vi "Map Child Elements.vi"(8 "error in":errorcluster, 10 "Address":i32[](array[numeric]), 11 "XML Document in":refnum<class "XML Document.lvclass">) -> (0 "error out":errorcluster, 3 "XML Document out":refnum<class "XML Document.lvclass">)   [LabVIEW 2014, in "XML Document.lvclass"]
uses:
  XML Document.lvclass
  Controls/Node Type.ctl
  Node_class/Node.lvclass
  <vilib>/xml/Close Reference(Node).vi
  <resource>/objmgr/DOMUserDefRef.rc
  Element_class/Element.lvclass
  Text Node_class/Text Node.lvclass
  Comment Node_class/Comment Node.lvclass
  <vilib>/xml/NI_XML.lvlib
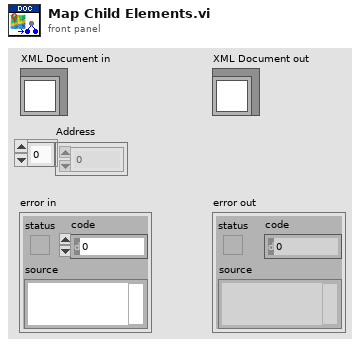
[diagram p1: front panel]
types:
  T1 = typedef "Node Type.ctl" = i32
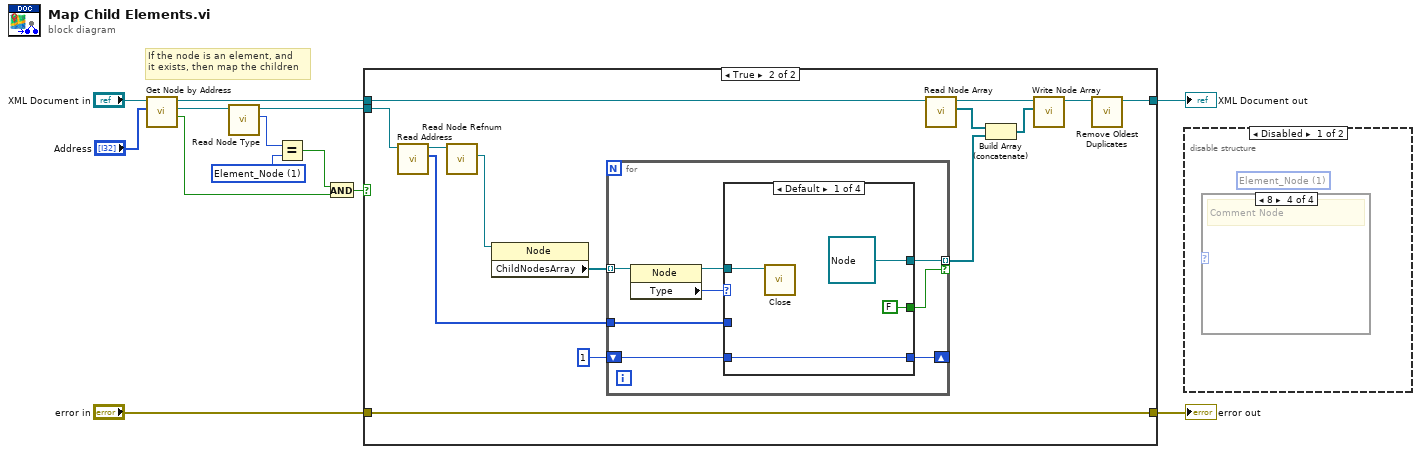
[diagram p0: block diagram]
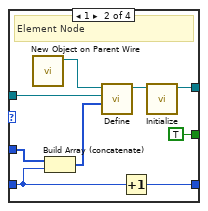
[diagram p7: hidden frame]
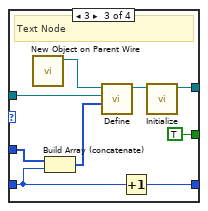
[diagram p8: hidden frame]
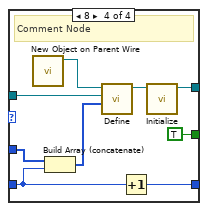
[diagram p9: hidden frame]
diagram:
  w4 = T1 1 items=["Element_Node"=1, "Attribute_Node"=2, "Text_Node"=3, "CDATASection_Node"=4, "EntityReference_Node"=5, "Entity_Node"=6, "ProcessingInstruction_Node"=7, "Comment_Node"=8, "Document_Node"=9, "DocumentType_Node"=10, "DocumentFragment_Node"=11, "Notation_Node"=12] ("y")
  # "If the node is an element, and\nit exists, then map the children"
  n1 = call "Get Node by Address.vi"("Address"="Address", "XML Document in"="XML Document in") -> ("Found?"=w3:bool, "Node.lvclass"=w9:refnum<class "Node.lvclass">, "XML Document out"=w10:refnum<class "XML Document.lvclass">)  [unwired: 6 in, 1 out]
  n2 = call-dynamic "Read Node Type.vi"("Node in"=w9) -> ("Node Type"=w5:T1, "Node out"=w6:refnum<class "Node.lvclass">)  [unwired: 8 in, 1 out]
  n3 = Equal?(x=w5, y=w4) -> (x = y?=w2:bool)
  n4 = And(x=w2, y=w3) -> (x .and. y?=w1:bool)
  n5 = case shown="True" w1 {
    tunnel: w10 -> [w15 w24]
    tunnel: w6 -> [_ w23]
    tunnel: [w15 w19] -> w12
    tunnel: "error in" -> [w14 w20]
    tunnel: [w14 w20] -> w7
    frame False {
    }
    frame True {
      n6 = call-dynamic "Read Address.vi"("Node in"=w23) -> ("Address"=w26:i32[], "Node out"=w27:refnum<class "Node.lvclass">)  [unwired: 8 in, 1 out]
      n7 = call-dynamic "Read Node Refnum.vi"("Node in"=w27) -> ("Node Refnum"=w29:refnum<k20>)  [unwired: 8 in, 2 out]
      n8 = property class="Node"(reference=w29) -> ("ChildNodesArray"=w28:refnum<k20>[])  [unwired: 1 in, 2 out]
      n9 = for {
        tunnel: w28 -> [w37] mode=indexing
        tunnel: w26 -> [w33]
        shift-right: [w32] -> _
        shift-left: 1 ("Address Location Part") -> [w34]
        tunnel: [w31] -> w17 mode=indexing if=w30
        n10 = property class="Node"(reference=w37) -> (reference out=w35:refnum<k20>, "Type"=w36:i32)  [unwired: 1 in, 1 out]
        n11 = case shown="Default" w36 {
          tunnel: w35 -> [w38 w47 w56 w65]
          tunnel: w34 -> [w41 w49 w58 w67]
          tunnel: w33 -> [_ w50 w59 w68]
          tunnel: [w41 w48 w57 w66] -> w32
          tunnel: [refnum<class "Node.lvclass"> refnum ("Node out") w42 w52 w61] -> w31
          tunnel: [FALSE TRUE TRUE TRUE] -> w30
          frame Default {
            n12 = call-poly <vilib>:"Close.vi"("node"=w38) -> ()  [unwired: 8 in, 1 out]
          }
          frame 1 {
            # "Element Node"
            n13 = call "New Object on Parent Wire.vi"() -> ("Node.lvclass"=w45:refnum<class "Node.lvclass">)  [unwired: 10 in, 1 out]
            n14 = Build Array (concatenate)(w50, w49) -> (w46:i32[])
            n15 = call-dynamic "Define.vi"("Address"=w46, "Node Refnum"=w47, "Node in"=w45) -> ("Node out"=w44:refnum<class "Node.lvclass">)  [unwired: 7 in, 1 out]
            n16 = Increment(x=w49) -> (x+1=w48:i32)
            n17 = call-dynamic "Initialize.vi"("Node in"=w44) -> ("Node out"=w42:refnum<class "Node.lvclass">)  [unwired: 9 in, 1 out]
          }
          frame 3 {
            # "Text Node"
            n18 = call "New Object on Parent Wire.vi"() -> ("Node.lvclass"=w54:refnum<class "Node.lvclass">)  [unwired: 10 in, 1 out]
            n19 = Build Array (concatenate)(w59, w58) -> (w55:i32[])
            n20 = call-dynamic "Define.vi"("Address"=w55, "Node Refnum"=w56, "Node in"=w54) -> ("Node out"=w53:refnum<class "Node.lvclass">)  [unwired: 7 in, 1 out]
            n21 = Increment(x=w58) -> (x+1=w57:i32)
            n22 = call-dynamic "Initialize.vi"("Node in"=w53) -> ("Node out"=w52:refnum<class "Node.lvclass">)  [unwired: 9 in, 1 out]
          }
          frame 8 {
            # "Comment Node"
            n23 = call "New Object on Parent Wire.vi"() -> ("Node.lvclass"=w63:refnum<class "Node.lvclass">)  [unwired: 10 in, 1 out]
            n24 = Build Array (concatenate)(w68, w67) -> (w64:i32[])
            n25 = call-dynamic "Define.vi"("Address"=w64, "Node Refnum"=w65, "Node in"=w63) -> ("Node out"=w62:refnum<class "Node.lvclass">)  [unwired: 7 in, 1 out]
            n26 = Increment(x=w67) -> (x+1=w66:i32)
            n27 = call-dynamic "Initialize.vi"("Node in"=w62) -> ("Node out"=w61:refnum<class "Node.lvclass">)  [unwired: 9 in, 1 out]
          }
        }
      }
      n28 = call-dynamic "Read Node Array.vi"("XML Document in"=w24) -> ("Node Array"=w18:refnum<class "Node.lvclass">[], "XML Document out"=w22:refnum<class "XML Document.lvclass">)  [unwired: 8 in, 1 out]
      n29 = Build Array (concatenate)(w18, w17) -> (w16:refnum<class "Node.lvclass">[])
      n30 = call-dynamic "Write Node Array.vi"("Node Array"=w16, "XML Document in"=w22) -> ("XML Document out"=w21:refnum<class "XML Document.lvclass">)  [unwired: 8 in, 1 out]
      n31 = call "Remove Oldest Duplicates.vi"("XML Document in"=w21) -> ("XML Document out"=w19:refnum<class "XML Document.lvclass">)  [unwired: 9 in, 1 out]
    }
  }
  "error out" <- w7
  "XML Document out" <- w12
  n32 = disable-structure shown="Disabled" {
    frame Disabled {
      (unwired) 1 items=["Element_Node"=1, "Attribute_Node"=2, "Text_Node"=3, "CDATASection_Node"=4, "EntityReference_Node"=5, "Entity_Node"=6, "ProcessingInstruction_Node"=7, "Comment_Node"=8, "Document_Node"=9, "DocumentType_Node"=10, "DocumentFragment_Node"=11, "Notation_Node"=12] ("Node Type")
      n33 = case shown="8" {
        selector: _ -> [_ _ _ _]
        frame Default {
        }
        frame 1 {
          # "Element Node"
        }
        frame 3 {
          # "Text Node"
        }
        frame 8 {
          # "Comment Node"
        }
      }
    }
    frame Enabled {
    }
  }
